vi "задача 3.01.vi"() -> ()   [LabVIEW 2019]
uses:
  <vilib>/Utility/file.llb/Read Delimited Spreadsheet (I64).vi
  <vilib>/Utility/file.llb/Write Delimited Spreadsheet (I64).vi
panel:
  out "Path 2":path
  out "Path":path
  out "XY Graph":cluster{"all rows":i64[], "all rows":i64[]}[](graph)
  out "Waveform Chart":dbl(graph)
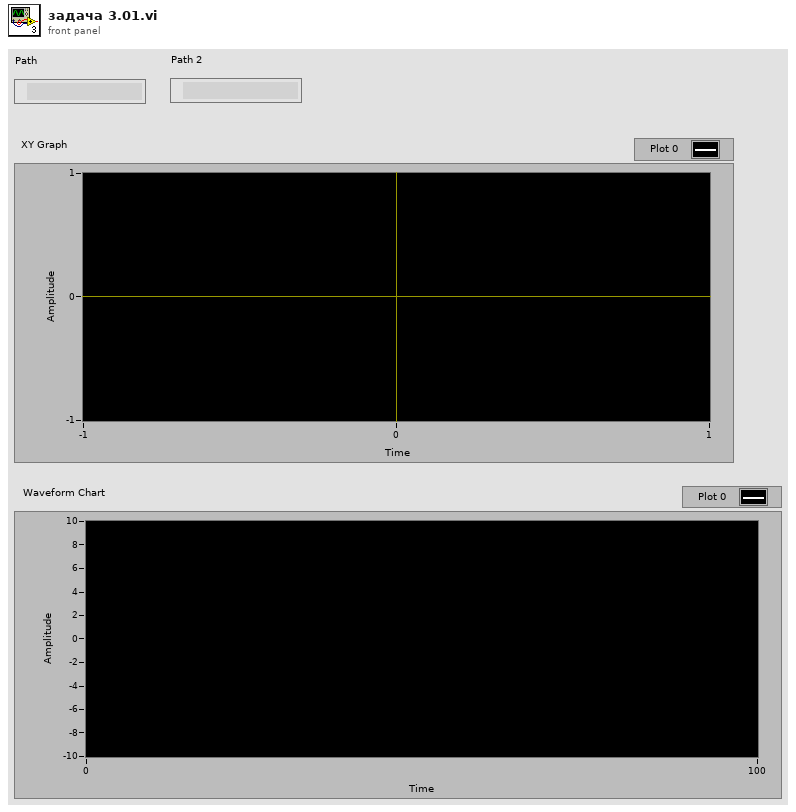
[diagram p1: front panel]
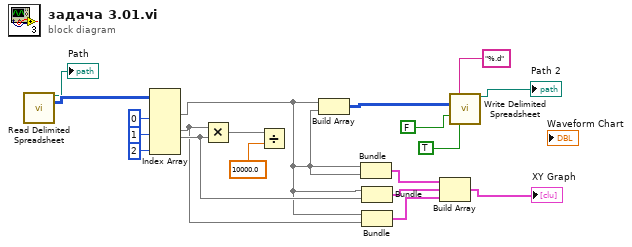
[diagram p0: block diagram]
diagram:
  n1 = call-poly <vilib>:"Read Delimited Spreadsheet.vi"() -> ("new file path (Not A Path if cancelled)"=→"Path":path, "all rows"=w19:i64[][])  [unwired: 10 in, 4 out]
  n2 = Index Array(array=w19, index (col) #1=0 ("disabled index (col)"), index (col) #2=1 ("index (col)"), index (col) #3=2 ("index (col)")) -> (element #1=w12:i64[], element #2=w11:i64[], element #3=w13:i64[])  [unwired: 3 in]
  n3 = Multiply(x=w11, y=w13) -> (x*y=w15:i64[])
  n4 = Divide(x=w15, y=10000.0) -> ()  [unwired: 1 out]
  n5 = Build Array(w12, w12) -> (w6:i64[][])
  n6 = Bundle("all rows"=w12, "all rows"=w12) -> (w10:cluster{"all rows":i64[], "all rows":i64[]})  [unwired: 1 in]
  n7 = Bundle("all rows"=w12, "all rows"=w13) -> (w9:cluster{"all rows":i64[], "all rows":i64[]})  [unwired: 1 in]
  n8 = Bundle("all rows"=w12, "all rows"=w11) -> (w8:cluster{"all rows":i64[], "all rows":i64[]})  [unwired: 1 in]
  n9 = Build Array(w10, w9, w8) -> (→"XY Graph":cluster{"all rows":i64[], "all rows":i64[]}[])
  n10 = call-poly <vilib>:"Write Delimited Spreadsheet.vi"("format (%d)"="%.d" ("format (%.3f)"), "2D data"=w6, "append to file? (new file:F)"=FALSE, "transpose? (no:F)"=TRUE) -> ("new file path (Not A Path if cancelled)"=→"Path 2":path)  [unwired: 10 in, 1 out]
